vi "mono_bbox.vi"(6 "python_parser_session":refnum<k35>, 7 "Sensor Connections":T1(array[cluster])) -> (0 "error out":errorcluster, 1 "python_session out":refnum<k35>, 2 "bbox_sample":T2, 3 "tcp_out":refnum<k5>)   [LabVIEW 2018, in "monoDrive.lvlib"]
uses:
  monoDrive.lvlib
panel:
  out "Sensor Connections Out":T1(array[cluster])
  out "size(s)":i32
  in  "mono_bbox_parser":path=path "C:/Users/celit/Documents/GitHub/client/lv_test.py"
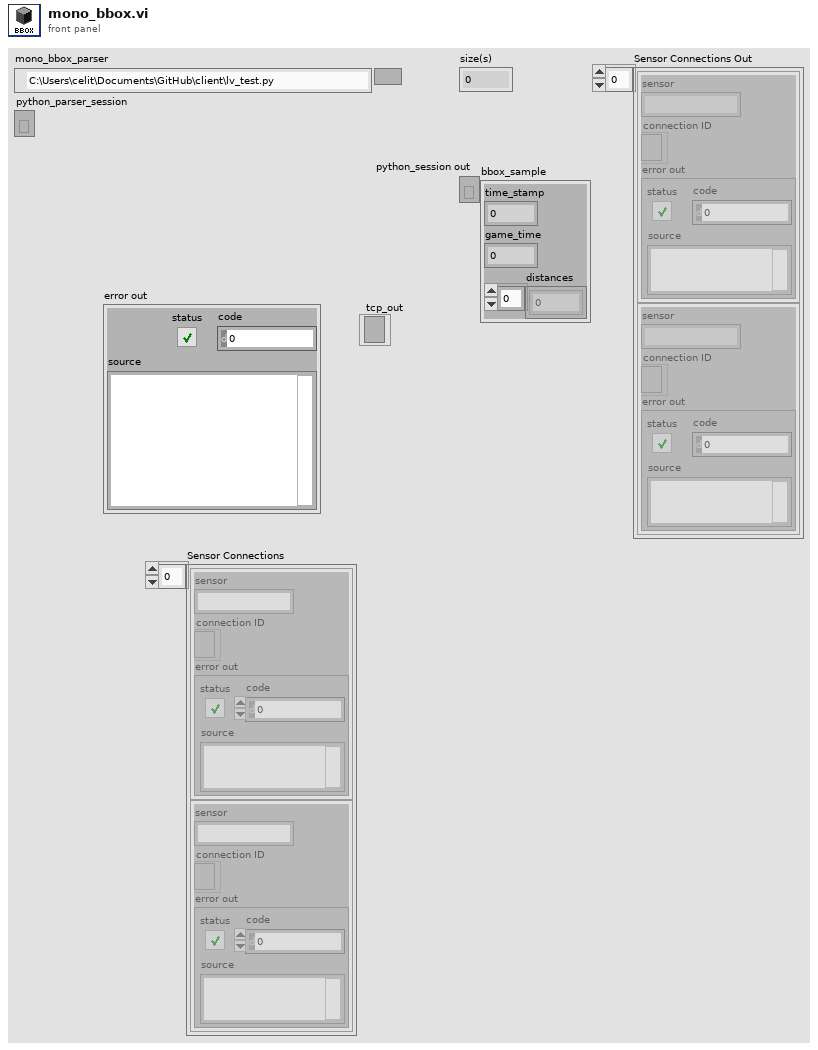
[diagram p1: front panel]
types:
  T1 = cluster{"sensor":string, "connection ID":refnum<k5>, "error out":errorcluster}[]
  T2 = cluster{"time_stamp":u32, "game_time":u32, "distances":sgl[]}
  T3 = cluster{"sensor":string, "connection ID":refnum<k5>, "error out":errorcluster}
  T4 = cluster{cluster{"length":u32, "time_stamp":u32, "game_time":sgl}, "data out":string}
  T5 = cluster{"length":u32, "time_stamp":u32, "game_time":sgl}
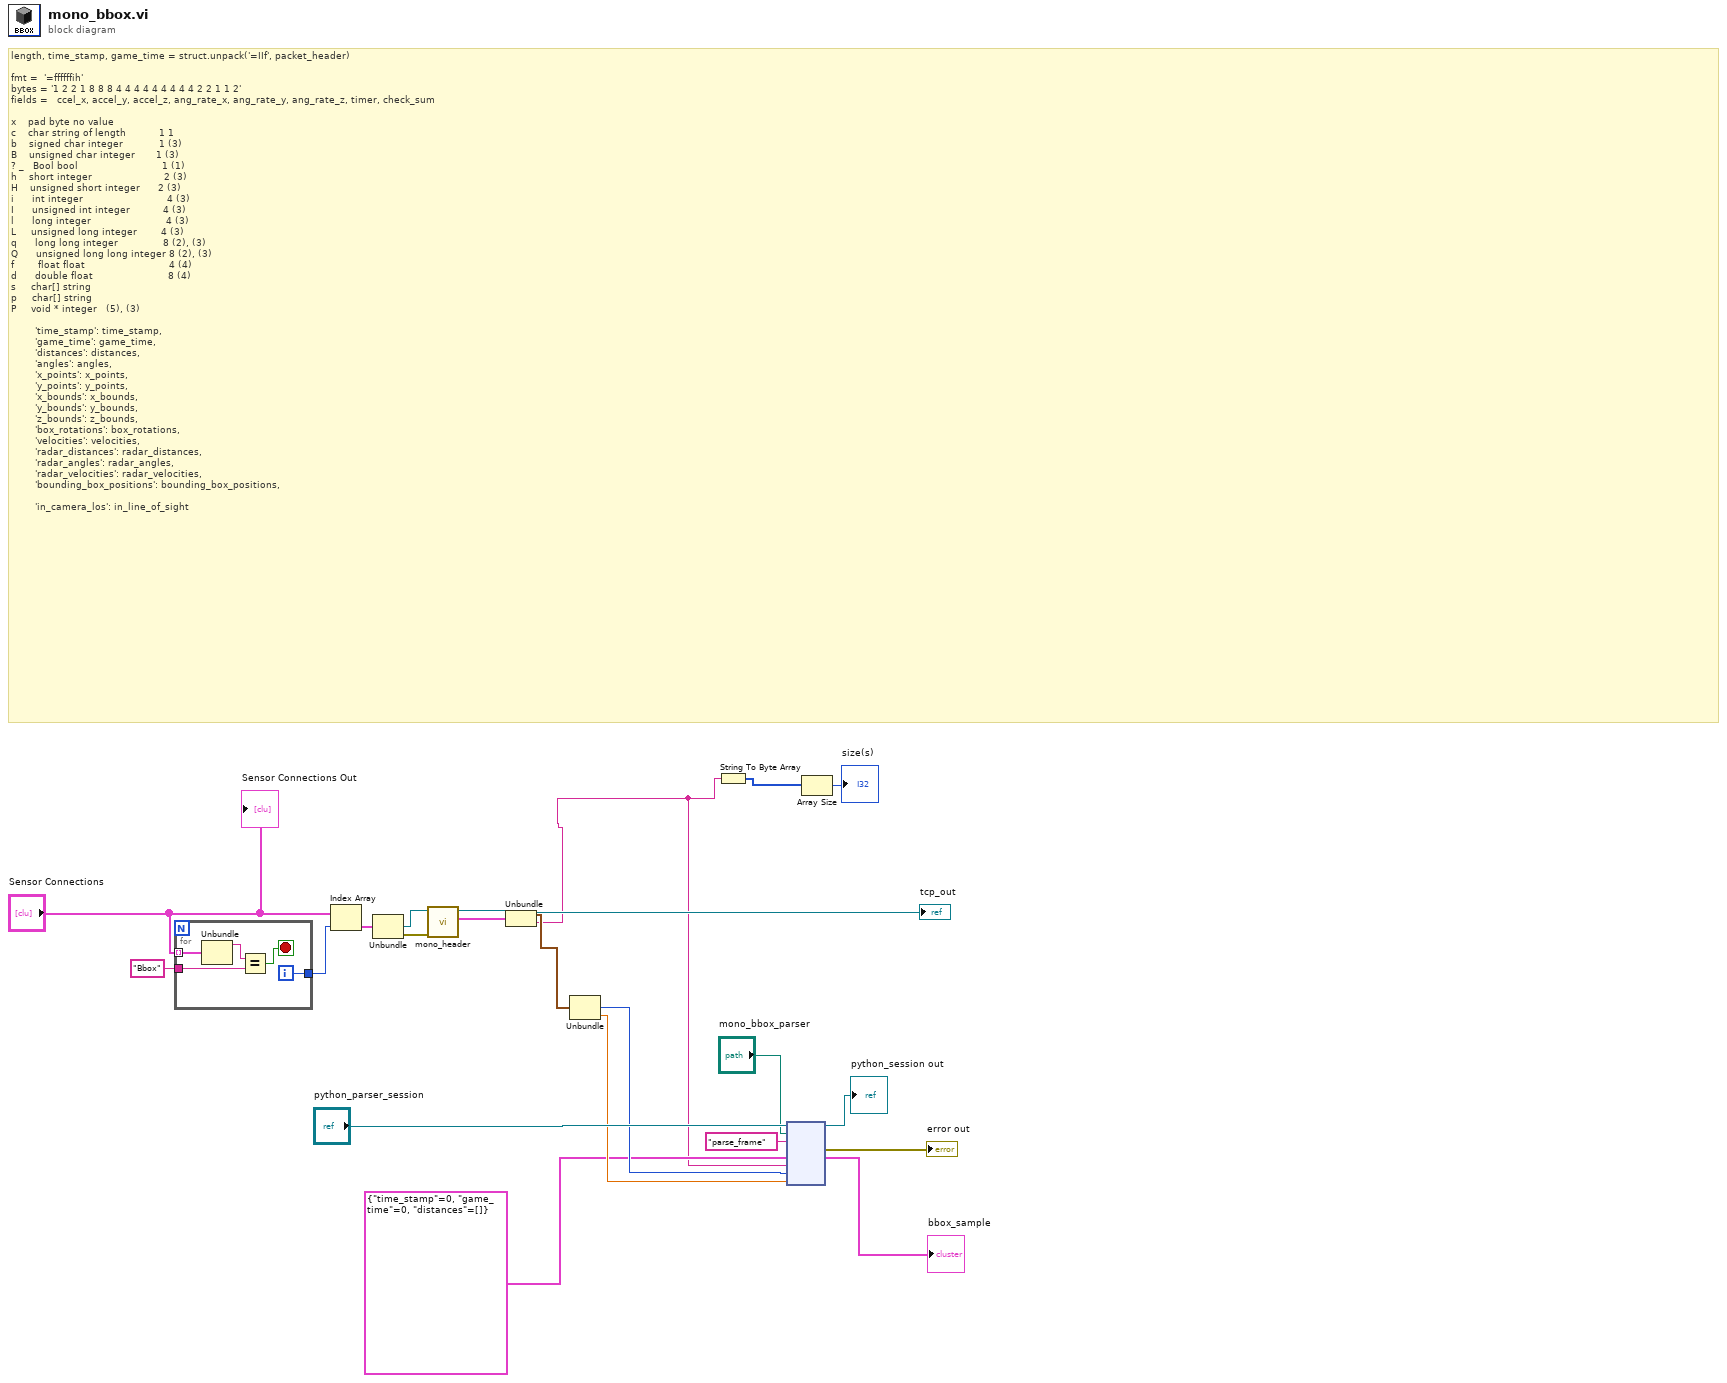
[diagram p0: block diagram]
diagram:
  # "length, time_stamp, game_time = struct.unpack('=IIf', packet_header)\n\nfmt =  '=ffffffih'\nbytes = '1 2 2 1 8 8 8 4 4 4 4 4 4 4 4 4 2 2 1 1 2'\nfields =   ccel_x, accel_y, accel_z, ang_rate_x, ang_rate_y, ang_rate_z, timer, check_sum\n\nx\t   pad byte\tno value\t \t \nc\t   char\tstring of length           1\t1\t \nb\t   signed char\tinteger\t           1\t(3)\nB\t   unsigned char\tinteger\t      1\t(3)\n?\t_   Bool\tbool\t                           1\t(1)\nh\t   short\tinteger\t                       2\t(3)\nH\t   unsigned short\tinteger\t     2\t(3)\ni\t     int\tinteger\t                           4\t(3)\nI\t     unsigned int\tinteger\t          4\t(3)\nl     \tlong\tinteger\t                        4\t(3)\nL\t    unsigned long\tinteger\t       4\t(3)\nq     \tlong long\tinteger\t              8\t(2), (3)\nQ\t     unsigned long long\tinteger\t8\t(2), (3)\nf       \tfloat\tfloat\t                           4\t(4)\nd     \tdouble\tfloat\t                        8\t(4)\ns\t    char[]\tstring\t \t \np\t    char[]\tstring\t \t \nP\t    void *\tinteger\t \t(5), (3)\n\n        'time_stamp': time_stamp,\n        'game_time': game_time,\n        'distances': distances,\n        'angles': angles,\n        'x_points': x_points,\n        'y_points': y_points,\n        'x_bounds': x_bounds,\n        'y_bounds': y_bounds,\n        'z_bounds': z_bounds,\n        'box_rotations': box_rotations,\n        'velocities': velocities,\n        'radar_distances': radar_distances,\n        'radar_angles': radar_angles,\n        'radar_velocities': radar_velocities,\n        'bounding_box_positions': bounding_box_positions,\n\n        'in_camera_los': in_line_of_sight"
  n1 = for {
    tunnel: "Sensor Connections" -> [w26] mode=indexing
    tunnel: "Bbox" -> [w24]
    tunnel: [w22] -> w16
    i -> [w22]
    stop <- w23 stop-if-true
    n2 = Unbundle(w26) -> ("sensor"=w25:string)  [unwired: 2 out]
    n3 = Equal?(x=w25, y=w24) -> (x = y?=w23:bool)
  }
  n4 = Index Array(array="Sensor Connections", index=w16) -> (element=w20:T3)
  n5 = Unbundle(w20) -> ("connection ID"=w18:refnum<k5>, "error out"=w17:errorcluster)  [unwired: 1 out]
  n6 = call "mono_header.vi"("error in"=w17, "connection ID"=w18) -> ("sensor_sample"=w21:T4, "connection ID out"=→"tcp_out":refnum<k5>)  [unwired: 7 in, 1 out]
  n7 = Unbundle(w21) -> (w11:T5, "data out"=w3:string)
  n8 = Unbundle(w11) -> ("time_stamp"=w9:u32, "game_time"=w10:sgl)  [unwired: 1 out]
  n9 = String To Byte Array(string=w3) -> (unsigned byte array=w2:u8[])
  n10 = node("python_parser_session", "mono_bbox_parser", "parse_frame" ("function name"), T2 {"time_stamp"=0, "game_time"=0, "distances"=[]}, w3, w9, w10) -> (→"python_session out":refnum<k35>, →"error out":errorcluster, →"bbox_sample":T2)  [unwired: 4 in, 2 out]
  n11 = Array Size(array=w2) -> (size(s)=→"size(s)":i32)
  "Sensor Connections Out" <- "Sensor Connections"
